vi "Daten Serialisieren - Linien Konfiguration.vi"(9 "Frame-ID":u32, 10 "Aktuelle Zeit":timestamp) -> (0 "Frame-ID letzter Wert":u32, 2 "data":T1[](array[typedef])=[{"timestamp"=timestamp(0 s since 1904-01-01), "payload"=[0, 2, 3, 4, 5, 6, 7, 8], "identifier"=2, "type"=0, "extended?"=FALSE, "echo?"=FALSE}, {"timestamp"=timestamp(0 s since 1904-01-01), "payload"=[0, 1, 2, 3, 4, 5, 6, 7], "identifier"=3, "type"=0, "extended?"=FALSE, "echo?"=FALSE}] {"payload" format="%x"; "timestamp" format="%<%.7X\n%x>T"; "type" items=["CAN Data"=0, "CAN Remote"=1, "CAN Bus Error"=2, "CAN 2.0 Data"=8, "CAN FD Data"=16, "CAN FD+BRS Data"=24, "J1939 Data"=192, "Delay"=224, "Log Trigger"=225, "Start Trigger"=226]; "identifier" format="%x"})   [LabVIEW 2020]
uses:
  <vilib>/xnet/xnet.llb/XNET Frame Type CAN.ctl
  <vilib>/xnet/xnet.llb/XNET Frame CAN.ctl
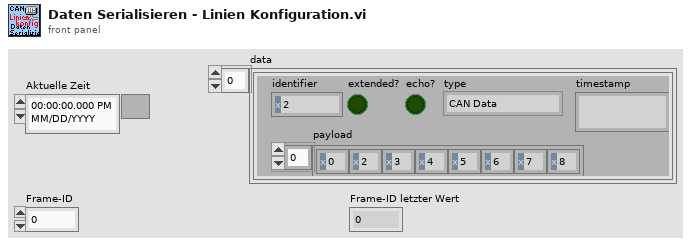
[diagram p1: front panel]
types:
  T1 = typedef "XNET Frame CAN.ctl" = cluster{"timestamp":timestamp, "payload":u8[], "identifier":u32, "type":T2, "extended?":bool, "echo?":bool}
  T2 = typedef "XNET Frame Type CAN.ctl" = u8
  T3 = typedef "Anlagenübersicht.lvlib/FGV Linienkonfiguration Aktionen.ctl" = enum16{"lesen", "Linie", "laden", "speichern"}
  T4 = typedef "Anlagenübersicht.lvlib/Linienkonfiguration.ctl" = cluster{"Linienkonfig Motor":T5, "Linienkonfig Container":T6, "Linienkonfig Motor 2":T5, "Linienkonfig Container 2":T6, "Linienkonfig Motor 3":T5, "Linienkonfig Container 3":T6}
  T5 = typedef "Anlagenübersicht.lvlib/Linienkonfiguration Motor.ctl" = enum8{"---", "VDOC", "NDOC", "NDPF", "NSCR", "Sonderpos."}
  T6 = typedef "Anlagenübersicht.lvlib/Linienkonfiguration Container_Array.ctl" = T7[]
  T7 = typedef "Anlagenübersicht.lvlib/Linienkonfiguration Container.ctl" = enum8{"---", "MSS-1", "MSS-2", "MSS-3", "FTIR-1", "FTIR-2", "FTIR-3", "PEG-1", "PEG-2", "PEG-3", "SEM-1", "SEM-2", "Sondermess."}
  T8 = enum16{"big-endian, network order", "native, host order", "little-endian"}
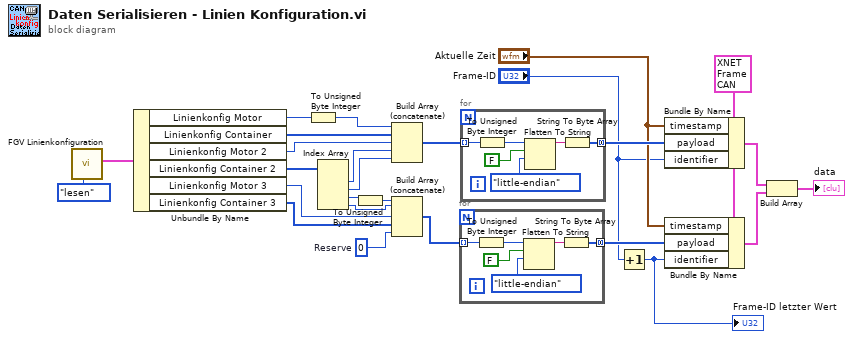
[diagram p0: block diagram]
diagram:
  w24 = T1 {"timestamp"=timestamp(0 s since 1904-01-01), "payload"=[0, 2, 3, 4, 5, 6, 7, 8], "identifier"=2, "type"=0, "extended?"=FALSE, "echo?"=FALSE} ("CAN frame")
  w19 = u8 0  # Reserve
  n1 = call "FGV Linienkonfiguration.vi"("Aktionen"=FGV_Linienkonfiguration_Aktionen."lesen") -> ("Linienkonfiguration"=w6:T4)  [unwired: 10 in]
  n2 = Unbundle By Name(w6) -> ("Linienkonfig Motor"=w8:T5, "Linienkonfig Container"=w10:T6, "Linienkonfig Motor 2"=w11:T5, "Linienkonfig Container 2"=w7:T6, "Linienkonfig Motor 3"=w17:T5, "Linienkonfig Container 3"=w18:T6)
  n3 = To Unsigned Byte Integer(number=w8) -> (unsigned 8bit integer=w9:u8)
  n4 = Index Array(array=w7) -> (element #1=w12:T7, element #2=w13:T7, element #3=w15:T7, element #4=w16:T7)  [unwired: 4 in]
  n5 = To Unsigned Byte Integer(number=w15) -> (unsigned 8bit integer=w14:u8)
  n6 = Build Array (concatenate)(w9, w10, w11, w12, w13) -> (w20:u8[])
  n7 = Build Array (concatenate)(w14, w16, w17, w18, w19) -> (w21:u8[])
  n8 = for {
    tunnel: w21 -> [w29] mode=indexing
    tunnel: [w28] -> w23 mode=concatenating
    n9 = To Unsigned Byte Integer(number=w29) -> (unsigned 8bit integer=w32:u8)
    n10 = Flatten To String(anything=w32, prepend array or string size? (T)=FALSE ("Array- oder String-Größe voranstellen? (T)"), byte order (0:big-endian, network order)=T8."little-endian" ("Byte-Reihenfolge (0:Big-Endian, Netzwerkreihenfolge)")) -> (data string=w30:string)  [unwired: 1 in, 2 out]
    n11 = String To Byte Array(string=w30) -> (unsigned byte array=w28:u8[])
  }
  n12 = for {
    tunnel: w20 -> [w35] mode=indexing
    tunnel: [w34] -> w22 mode=concatenating
    n13 = To Unsigned Byte Integer(number=w35) -> (unsigned 8bit integer=w38:u8)
    n14 = Flatten To String(anything=w38, prepend array or string size? (T)=FALSE ("Array- oder String-Größe voranstellen? (T)"), byte order (0:big-endian, network order)=T8."little-endian" ("Byte-Reihenfolge (0:Big-Endian, Netzwerkreihenfolge)")) -> (data string=w36:string)  [unwired: 1 in, 2 out]
    n15 = String To Byte Array(string=w36) -> (unsigned byte array=w34:u8[])
  }
  n16 = Increment(x="Frame-ID") -> (x+1=w1:u32)
  "Frame-ID letzter Wert" <- w1
  n17 = Bundle By Name(cluster=w24, "timestamp"="Aktuelle Zeit", "payload"=w22, "identifier"="Frame-ID") -> (w25:T1)
  n18 = Bundle By Name(cluster=w24, "timestamp"="Aktuelle Zeit", "payload"=w23, "identifier"=w1) -> (w26:T1)
  n19 = Build Array(w25, w26) -> (→"data":T1[])
